vi "MaxiGauge_get_status.vi"() -> ()   [LabVIEW 2019]
panel:
  out "Output 2":string
  in  "Delay":u32=500
  in  "VISA resource name":refnum<visa-resource-name>
  out "Output":string
  # "Should return <ACK><CR><LF>"
  # "Should return sensor 1-6 status <CR><LF>"
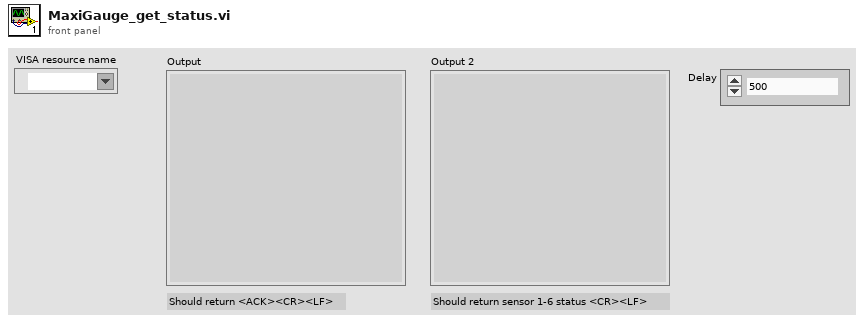
[diagram p1: front panel]
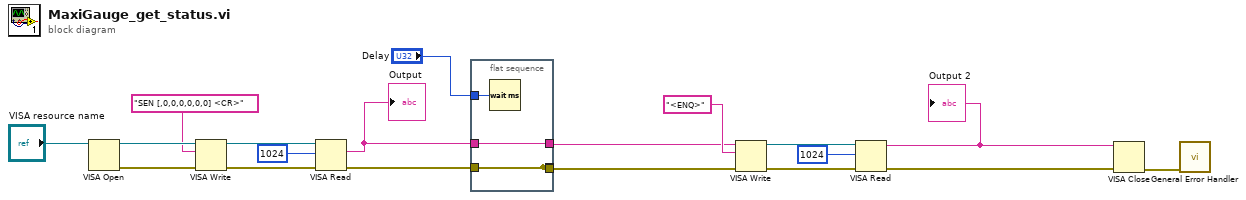
[diagram p0: block diagram]
diagram:
  n1 = VISA Open(VISA resource name="VISA resource name") -> (VISA resource name=w18:refnum<visa-resource-name>, error out=w15:errorcluster)  [unwired: 4 in]
  n2 = VISA Write(VISA resource name=w18, write buffer="SEN [,0,0,0,0,0,0] <CR>" ("String"), error in (no error)=w15) -> (VISA resource name out=w17:refnum<visa-resource-name>, error out=w14:errorcluster)  [unwired: 1 out]
  n3 = VISA Read(VISA resource name=w17, byte count=u32 1024 ("unsigned 32bit integer"), error in (no error)=w14) -> (read buffer=w11:string, error out=w10:errorcluster)  [unwired: 2 out]
  "Output" <- w11
  n4 = flat-sequence {
    tunnel: w10 -> [w20]
    tunnel: [w20] -> _
    tunnel: w11 -> [w21]
    tunnel: [w21] -> w2
    tunnel: "Delay" -> [w22]
    tunnel: [w20] -> w1
    frame #0 {
      n5 = Wait (ms)(milliseconds to wait=w22) -> ()  [unwired: 1 out]
    }
  }
  n6 = VISA Write(VISA resource name=w2, write buffer="<ENQ>" ("String"), error in (no error)=w1) -> (VISA resource name out=w8:refnum<visa-resource-name>, error out=w6:errorcluster)  [unwired: 1 out]
  n7 = VISA Read(VISA resource name=w8, byte count=u32 1024 ("unsigned 32bit integer"), error in (no error)=w6) -> (read buffer=w4:string, error out=w3:errorcluster)  [unwired: 2 out]
  "Output 2" <- w4
  n8 = VISA Close(VISA resource name=w4, error in (no error)=w3) -> (error out=w9:errorcluster)
  n9 = call <vilib>:"General Error Handler.vi"("error in (no error)"=w9) -> ()  [unwired: 10 in, 5 out]
